vi "DrawCircleVision.vi"() -> ()   [LabVIEW 2019]
uses:
  <vilib>/userDefined/High Color/IMAQdx.ctl
panel:
  out "CenterYmmGH":dbl
  out "CenterXmmGH":dbl
  out "Thickness(um)":dbl
  out "OuterRadius(um)":dbl
  out "InnerRadius(um)":dbl
  in  "microns/pixel":dbl=0.4348 format="%#_13g"
  out "Image 3":T1(plugin-control)
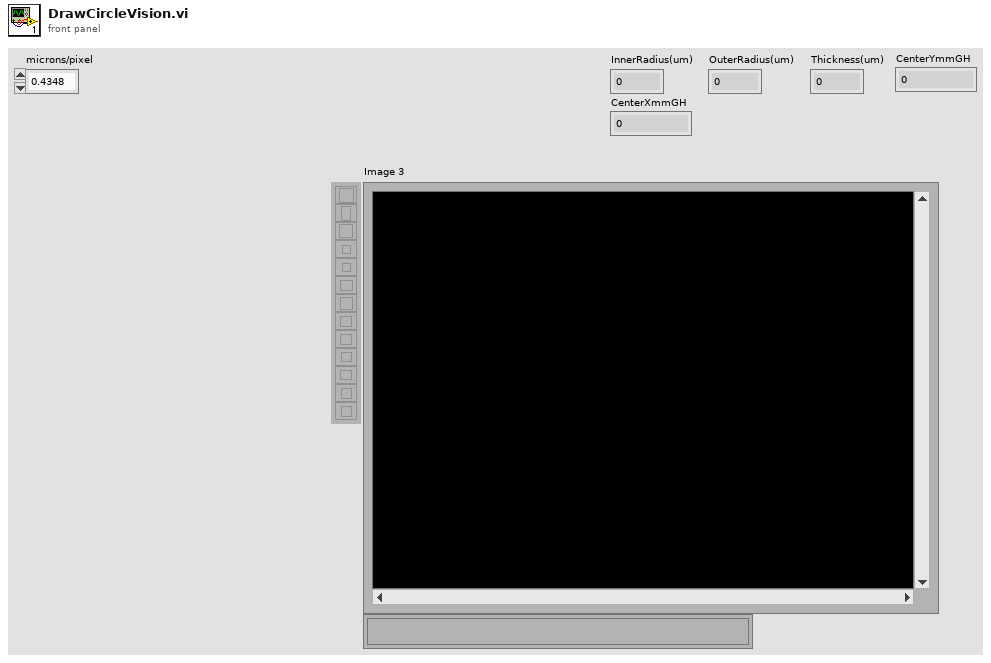
[diagram p1: front panel]
types:
  T1 = typedef "IMAQ Image.ctl" = refnum<image>
  T2 = typedef "IMAQdx.ctl" = refnum<k21>
  T3 = typedef "IMAQ Circle" = cluster{"Center X":i32, "Center Y":i32, "Inner Radius":i32, "Outer Radius":i32, "Start Angle":dbl, "End Angle":dbl}
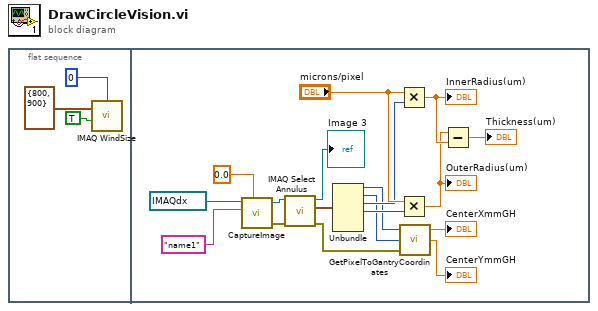
[diagram p0: block diagram]
diagram:
  n1 = flat-sequence {
    frame #0 {
      n2 = call "IMAQ WindSize"("Scrollbars? (N)"=TRUE, "Width & Height"=cluster{"Width":i32, "Height":i32} {"Width"=800, "Height"=900}, "Window Number"=0) -> ()  [unwired: 3 in, 3 out]
    }
    frame #1 {
      n3 = call "CaptureImage.vi"("Camera"=T2 "cam0", "Rotate (degrees)"=sgl 0.0, "ImageName"="name1") -> ("Image"=w8:T1, "error out"=w9:errorcluster)  [unwired: 4 in]
      n4 = call "IMAQ Select Annulus"("error in (no error)"=w9, "Image In"=w8) -> ("error out"=w14:errorcluster, "Annulus"=w10:T3, "Image Out (duplicate)"=→"Image 3":T1)  [unwired: 6 in, 1 out]
      n5 = Unbundle(w10) -> ("Center X"=w12:i32, "Center Y"=w13:i32, "Inner Radius"=w15:i32, "Outer Radius"=w16:i32)  [unwired: 2 out]
      n6 = Multiply(x="microns/pixel", y=w15) -> (x*y=w19:dbl)
      "InnerRadius(um)" <- w19
      n7 = Multiply(x="microns/pixel", y=w16) -> (x*y=w18:dbl)
      "OuterRadius(um)" <- w18
      n8 = call "GetPixelToGantryCoordinates.vi"("error in (no error)"=w14, "PixelY"=w13, "PixelX"=w12) -> ("YmmGH"=→"CenterYmmGH":dbl, "XmmGH"=→"CenterXmmGH":dbl)  [unwired: 1 out]
      n9 = Subtract(x=w18, y=w19) -> (x-y=→"Thickness(um)":dbl)
    }
  }
